vi "LJT4_extract_TC_V.vi"(4 "amp_gain":dbl[](array[numeric])=[261.0, 261.0, 261.0, 261.0], 6 "amp_offset":dbl[](array[numeric])=[1.25, 1.25, 1.235, 1.254], 7 "chan":i32[](array[numeric])=[4, 5, 6, 7], 11 "voltage_raw":dbl[](array[numeric])) -> (0 "voltage_raw_out":dbl[](array[numeric]), 3 "voltage_TC":dbl[](array[numeric]))   [LabVIEW 2019]
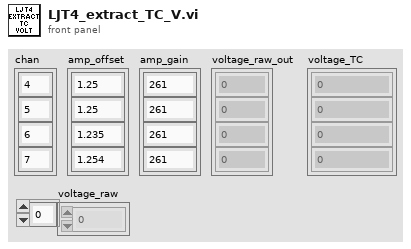
[diagram p1: front panel]
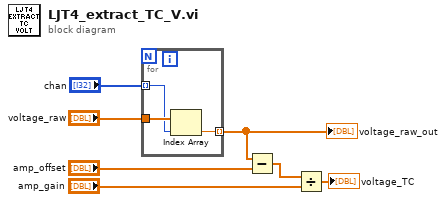
[diagram p0: block diagram]
diagram:
  n1 = for {
    tunnel: "voltage_raw" -> [w10]
    tunnel: "chan" -> [w9] mode=indexing
    tunnel: [w8] -> w5 mode=indexing
    n2 = Index Array(array=w10, index=w9) -> (element=w8:dbl)
  }
  "voltage_raw_out" <- w5
  n3 = Subtract(x=w5, y="amp_offset") -> (x-y=w3:dbl[])
  n4 = Divide(x=w3, y="amp_gain") -> (x/y=→"voltage_TC":dbl[])
